vi "Get 1D I64.vi"(5 "format string (%_20f)":string="%_20f", 7 "key description":string, 8 "sections":string[](array[string]), 9 "numeric":i64[](array[numeric]), 11 "info data":string) -> (0 "sections out":string[](array[string]), 1 "found?":bool, 2 "value":i64[](array[numeric]), 3 "info data out":string)   [LabVIEW 2013, in "infolib.lvlib"]
doc: "Add a new numeric key to Info Data string. If section exists in Info Data string, inserts key into this section."
uses:
  infolib.lvlib
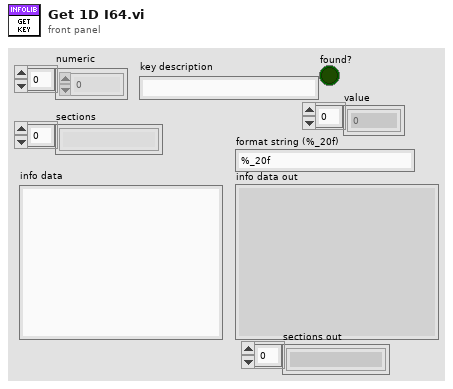
[diagram p1: front panel]
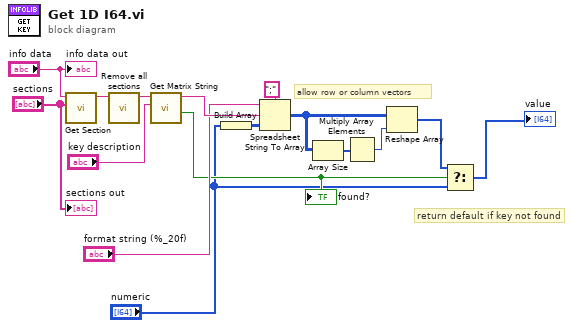
[diagram p0: block diagram]
diagram:
  # "return default if key not found"
  # "allow row or column vectors"
  n1 = call "Get Section.vi"("sections"="sections", "info data"="info data") -> ("section part"=w16:string)  [unwired: 8 in, 1 out]
  n2 = call "Remove all sections.vi"("info data"=w16) -> ("info data out"=w13:string)  [unwired: 10 in]
  n3 = call "Get Matrix String.vi"("matrix key"="key description", "info data"=w13) -> ("exist"=w4:bool, "matrix part"=w11:string)  [unwired: 8 in]
  "found?" <- w4
  n4 = Build Array("numeric") -> (w5:i64[][])
  n5 = Spreadsheet String To Array(delimiter (Tab)=";", format string="format string (%_20f)", spreadsheet string=w11, array type (2D Dbl)=w5) -> (array=w6:i64[][])
  n6 = Array Size(array=w6) -> (size(s)=w8:i32[])
  n7 = Multiply Array Elements(1:w8) -> (0:w7:i32)
  n8 = Reshape Array(w6, w7) -> (w2:i64[])
  n9 = Select(t=w2, s=w4, f="numeric") -> (s? t:f=→"value":i64[])
  "info data out" <- "info data"
  "sections out" <- "sections"
